vi "read_TCUStatus4.vi"(1 "Array":u8[](array[numeric])=[0, 0, 0, 0, 0, 0, 0, 0, 0, 0, 0, 0, 0, 0, 0, 0, 0, 0, 0, 0, 0, 0, 0, 0, 0, 0, 0, 0, 0, 0, 0, 0, 0, 0, 0, 0, 0, 0, 0, 0, 0, 0, 0, 0, 0, 0, 0, 0, 0, 0, 0, 0, 0, 0, 0, 0, 0, 0, 0, 0, 0, 0, 0, 0, 0, 0, 0, 0, 0, 0, 0, 0, 0, 0, 0, 0, 0, 0, 0, 0, 0, 0, 0, 0, 0, 0, 0, 0, 0, 0, 0, 0, 0, 0, 0, 0, 0, 0, 0, 0, 0, 0, 0, 0, 0, 0, 0, 0, 0, 0, 0, 0, 0, 0, 0, 0, 0, 0, 0, 0, 0, 0, 0, 0, 0, 0, 0, 0, 0, 0, 0, 0, 0, 0, 0, 0, 0, 0, 0, 0, 0, 0, 0, 0, 0, 0, 0, 0, 0, 0, 0, 0, 0, 0, 0, 0, 0, 0, 0, 0, 0, 0, 0, 0, 0, 0, 0, 0, 0, 0, 0, 0, 0, 0, 0, 0, 0, 0, 0, 0, 0]) -> (0 "Message":T1)   [LabVIEW 2017]
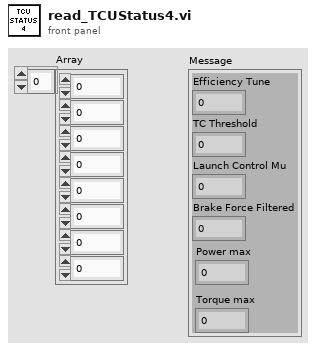
[diagram p1: front panel]
types:
  T1 = cluster{"Efficiency Tune":dbl, "TC Threshold":u8, "Launch Control Mu":dbl, "Brake Force Filtered":u16, "Power max":u8, "Torque max":u8}
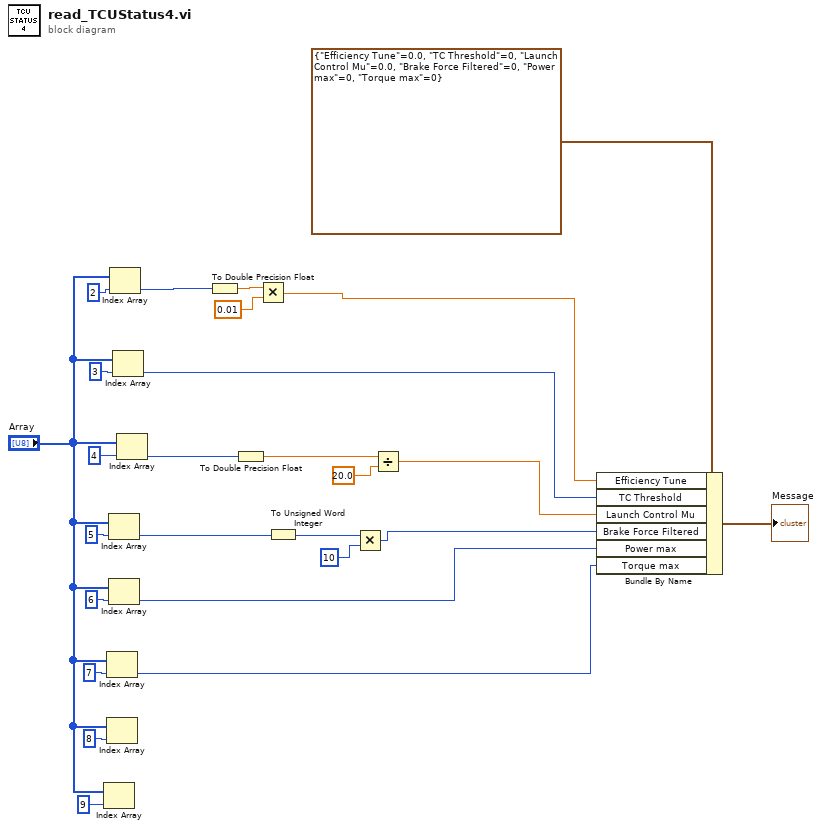
[diagram p0: block diagram]
diagram:
  n1 = Index Array(array="Array", index=9) -> ()  [unwired: 1 out]
  n2 = Index Array(array="Array", index=7) -> (element=w1:u8)
  n3 = Index Array(array="Array", index=8) -> ()  [unwired: 1 out]
  n4 = Index Array(array="Array", index=5) -> (element=w5:u8)
  n5 = Index Array(array="Array", index=6) -> (element=w2:u8)
  n6 = Index Array(array="Array", index=2) -> (element=w14:u8)
  n7 = Index Array(array="Array", index=3) -> (element=w9:u8)
  n8 = Index Array(array="Array", index=4) -> (element=w12:u8)
  n9 = To Double Precision Float(number=w14) -> (double precision float=w16:dbl)
  n10 = To Double Precision Float(number=w12) -> (double precision float=w8:dbl)
  n11 = Multiply(x=w16, y=0.01) -> (x*y=w10:dbl)
  n12 = To Unsigned Word Integer(number=w5) -> (unsigned 16bit integer=w7:u16)
  n13 = Multiply(x=w7, y=u16 10) -> (x*y=w4:u16)
  n14 = Divide(x=w8, y=20.0) -> (x/y=w11:dbl)
  n15 = Bundle By Name(cluster=T1 {"Efficiency Tune"=0.0, "TC Threshold"=0, "Launch Control Mu"=0.0, "Brake Force Filtered"=0, "Power max"=0, "Torque max"=0}, "Efficiency Tune"=w10, "TC Threshold"=w9, "Launch Control Mu"=w11, "Brake Force Filtered"=w4, "Power max"=w2, "Torque max"=w1) -> (→"Message":T1)
